vi "Meas Result Generate TWM Digitizer Correction - Generate CSV Matrix.vi"(5 "comment":string, 6 "header":string, 7 "CSV path":path, 8 "error in (no error)":errorcluster, 9 "uncertainty":dbl[][](array[numeric]), 10 "data":dbl[][](array[numeric]), 11 "f [Hz]":dbl[](array[numeric])) -> (0 "error out":errorcluster)   [LabVIEW 2013]
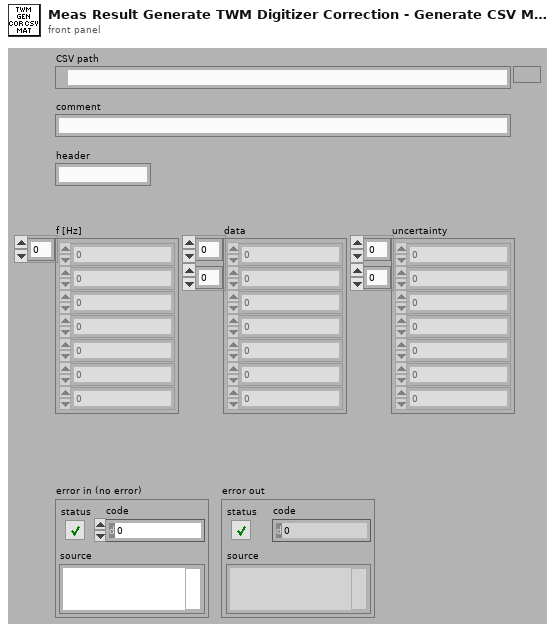
[diagram p1: front panel]
types:
  T1 = enum16{"open", "replace", "create", "open or create", "replace or create", "replace or create with confirmation"}
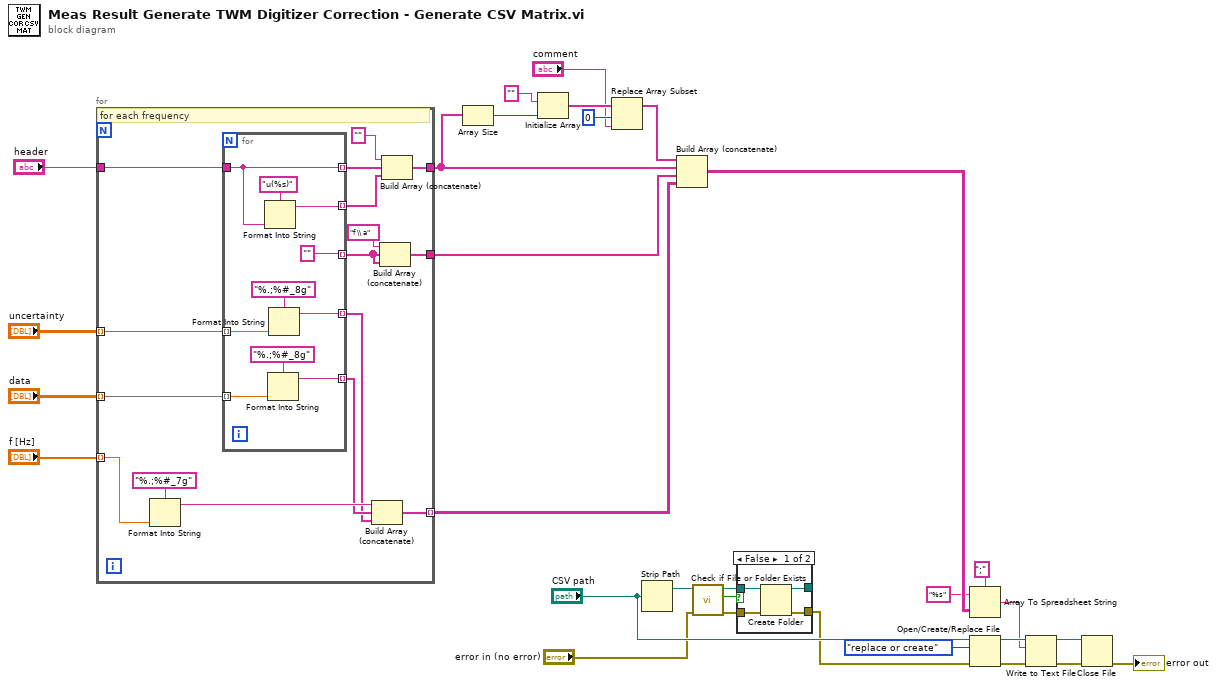
[diagram p0: block diagram]
diagram:
  n1 = for {
    tunnel: "f [Hz]" -> [w44] mode=indexing
    tunnel: "data" -> [w46] mode=indexing
    tunnel: "uncertainty" -> [w43] mode=indexing
    tunnel: [w39] -> w18 mode=indexing
    tunnel: [w36] -> w19
    tunnel: "header" -> [w35]
    tunnel: [w31] -> w20
    # "for each frequency"
    n2 = Format Into String(format string="%.;%#_7g", w44) -> (resulting string=w42:string)  [unwired: 2 in, 1 out]
    n3 = for {
      tunnel: w46 -> [w55] mode=indexing
      tunnel: w43 -> [w53] mode=indexing
      tunnel: [w52] -> w40 mode=indexing
      tunnel: [w51] -> w41 mode=indexing
      tunnel: [""] -> w38 mode=indexing
      tunnel: w35 -> [w48]
      tunnel: [w48] -> w33 mode=indexing
      tunnel: [w47] -> w32 mode=indexing
      n4 = Format Into String(format string="u(%s)", w48) -> (resulting string=w47:string)  [unwired: 2 in, 1 out]
      n5 = Format Into String(format string="%.;%#_8g", w55) -> (resulting string=w51:string)  [unwired: 2 in, 1 out]
      n6 = Format Into String(format string="%.;%#_8g", w53) -> (resulting string=w52:string)  [unwired: 2 in, 1 out]
    }
    n7 = Build Array (concatenate)(w42, w41, w40) -> (w39:string[])
    n8 = Build Array (concatenate)("f \\ a", w38, w38) -> (w36:string[])
    n9 = Build Array (concatenate)("", w33, w32) -> (w31:string[])
  }
  n10 = Array Size(array=w20) -> (size(s)=w26:i32)
  n11 = Initialize Array("", w26) -> (w24:string[])
  n12 = Replace Array Subset(array=w24, new element="comment", index=0) -> (w21:string[])
  n13 = Strip Path(path="CSV path") -> (stripped path=w14:path)  [unwired: 1 out]
  n14 = Build Array (concatenate)(w21, w20, w19, w18) -> (w12:string[][])
  n15 = call <vilib>:"Check if File or Folder Exists.vi"("error in (no error)"="error in (no error)", "path"=w14) -> ("error out"=w15:errorcluster, "file or folder exists?"=w17:bool, "dup path"=w16:path)  [unwired: 7 in]
  n16 = case shown="False" w17 {
    tunnel: w16 -> [w60 w61]
    tunnel: [w59 w61] -> _
    tunnel: w15 -> [w58 w62]
    tunnel: [w57 w62] -> w8
    frame False {
      n17 = Create Folder(path (use dialog)=w60, error in=w58) -> (created path=w59:path, error out=w57:errorcluster)  [unwired: 1 in, 1 out]
    }
    frame True {
    }
  }
  n18 = Array To Spreadsheet String(delimiter (Tab)=";", array=w12, 3:"%s" ("format string")) -> (spreadsheet string=w4:string)
  n19 = Open/Create/Replace File(file path (use dialog)="CSV path", error in=w8, operation (0:open)=T1."replace or create") -> (refnum out=w5:refnum<file>, error out=w6:errorcluster)  [unwired: 3 in, 1 out]
  n20 = Write to Text File(file (use dialog)=w5, text=w4, error in=w6) -> (refnum out=w2:refnum<file>, error out=w3:errorcluster)  [unwired: 1 in, 1 out]
  n21 = Close File(refnum=w2, error in=w3) -> (error out=→"error out":errorcluster)  [unwired: 1 out]
